vi "Configure Trend Partial.vi"(0 "VISA resource name":refnum<visa-resource-name>, 5 "Enable Partial Expanded Display (Disable)":bool, 11 "error in (no error)":errorcluster) -> (4 "VISA resource name out":refnum<visa-resource-name>, 15 "error out":errorcluster)   [LabVIEW 2020, in "Yokogawa GX Series.lvlib"]
doc: "Sets enable or disable the partial expanded trend display.\n\nValid range: STrdPartial\n\nNote: This VI does nothing when the instrument is GM10."
uses:
  <instrlib>/Yokogawa GX Series/Yokogawa GX Series.lvlib
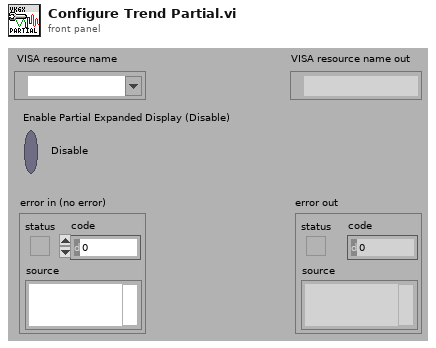
[diagram p1: front panel]
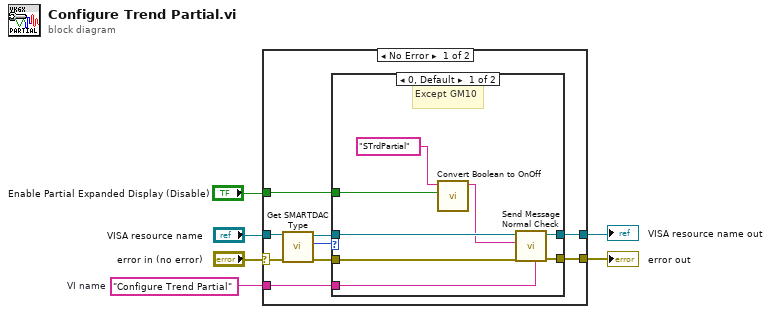
[diagram p0: block diagram]
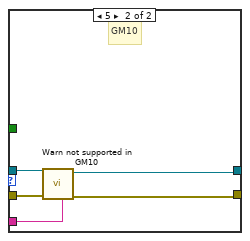
[diagram p2: hidden frame]
diagram:
  w5 = "Configure Trend Partial"  # VI name
  n1 = case shown="No Error" "error in (no error)" {
    selector: "error in (no error)" -> [w10 w29]
    tunnel: "VISA resource name" -> [w11 w30]
    tunnel: w5 -> [w15 _]
    tunnel: [w14 w30] -> w4
    tunnel: [w13 w29] -> w3
    tunnel: "Enable Partial Expanded Display (Disable)" -> [w12 _]
    frame No Error {
      n2 = call <instrlib>:"Get SMARTDAC Type.vi"("error in (no error)"=w10, "VISA resource name"=w11) -> ("error out"=w8:errorcluster, "SMARTDAC+ Type"=w7:u16, "VISA resource name out"=w9:refnum<visa-resource-name>)  [unwired: 7 in]
      n3 = case shown="0, Default" w7 {
        tunnel: w9 -> [w23 w28]
        tunnel: w15 -> [w22 w24]
        tunnel: [w21 w26] -> w14
        tunnel: [w20 w25] -> w13
        tunnel: w12 -> [w18 _]
        tunnel: w8 -> [w16 w27]
        frame 0, Default {
          # "Except GM10"
          n4 = call <instrlib>:"Convert Boolean to OnOff.vi"("On/Off"=w18, "Initial String (\"\")"="STrdPartial") -> ("Resulting String"=w17:string)  [unwired: 9 in]
          n5 = call <instrlib>:"Send Message Normal Check.vi"("Source (\"\")"=w22, "error in (no error)"=w16, "Send Message (\"\")"=w17, "VISA resource name"=w23) -> ("error out"=w20:errorcluster, "VISA resource name out"=w21:refnum<visa-resource-name>)  [unwired: 2 in, 4 out]
        }
        frame 5 {
          # "GM10"
          n6 = call <instrlib>:"Warn not supported in GM10.vi"("Source (\"\")"=w24, "error in (no error)"=w27, "VISA resource name"=w28) -> ("error out"=w25:errorcluster, "VISA resource name out"=w26:refnum<visa-resource-name>)  [unwired: 7 in]
        }
      }
    }
    frame Error {
    }
  }
  "error out" <- w3
  "VISA resource name out" <- w4
